vi "Bundle.vi"(8 "error in (no error)":errorcluster, 10 "Sub Panel":refnum<vi>, 11 "Manual Edit in":refnum<class "Manual Edit.lvclass">) -> (0 "error out":errorcluster, 3 "Manual Edit out":refnum<class "Manual Edit.lvclass">)   [LabVIEW 2020, in "Msg.lvlib" / "Manual Edit.lvclass"]
uses:
  Manual Edit.lvclass
  Manual Edit.lvclass/Manual Edit.ctl
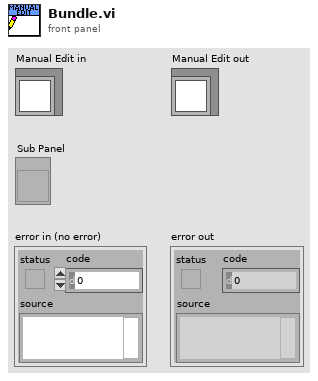
[diagram p1: front panel]
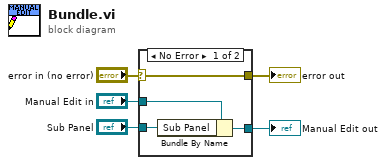
[diagram p0: block diagram]
diagram:
  n1 = case shown="No Error" "error in (no error)" {
    selector: "error in (no error)" -> [w9 w10]
    tunnel: [w9 w10] -> w4
    tunnel: [w7 w11] -> w2
    tunnel: "Manual Edit in" -> [w8 w11]
    tunnel: "Sub Panel" -> [w6 _]
    frame No Error {
      n2 = Bundle By Name(cluster=w8, "Sub Panel"=w6) -> (w7:refnum<class "Manual Edit.lvclass">)
    }
    frame Error {
    }
  }
  "error out" <- w4
  "Manual Edit out" <- w2
